vi "LVClass_WavefrontCorrectorSet Get Actions List.vi"(0 "WavefrontCorrectorSet in":refnum<class "WavefrontCorrectorSet.lvclass">, 11 "error in (no error)":errorcluster) -> (4 "WavefrontCorrectorSet out":refnum<class "WavefrontCorrectorSet.lvclass">, 6 "Actions list":string[](array[string]), 15 "error out":errorcluster)   [LabVIEW 2020, in "WavefrontCorrectorSet.lvclass"]
doc: "If parameter is a string to be selected among a finite set of strings, return\nthe size of this set. See Imop_WavefrontCorrectorSet_GetParameterOption.\n\n--------------------------------------------------------------------------------\n\n<B>wavefrontcorrector_setIn </B> : WavefrontCorrectorSet object.\n<B>wavefrontcorrector_setOut </B> : WavefrontCorrectorSet object.\n<B>parameter_name </B> : Parameter name.\n<B>size </B> : Size of the list (count of strings expected in that parameter).\n<B>ErrorIn </B> : Error\n<B>ErrorOut </B> : Error\n\n--------------------------------------------------------------------------------"
uses:
  WavefrontCorrectorSet.lvclass
  WavefrontCorrectorSet.lvclass/WavefrontCorrectorSet.ctl
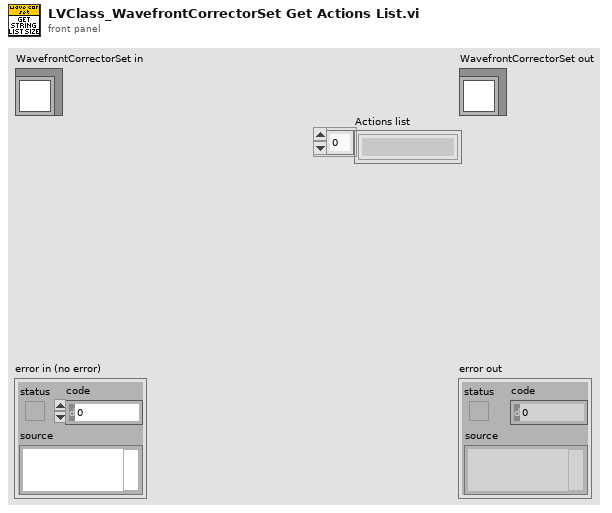
[diagram p1: front panel]
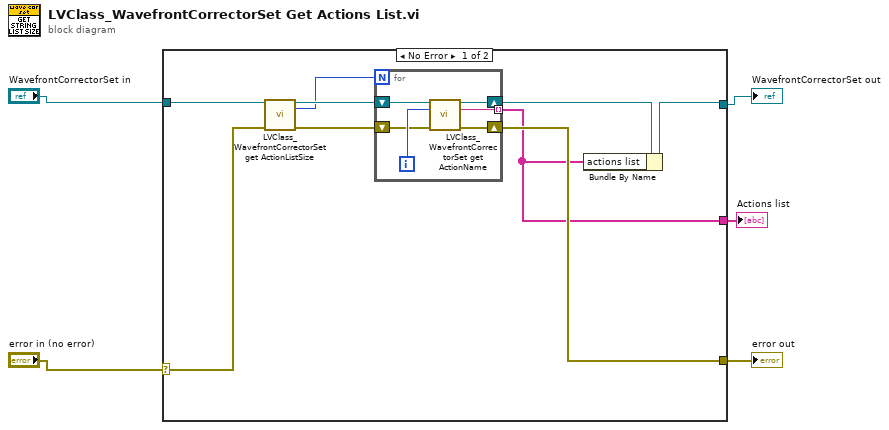
[diagram p0: block diagram]
diagram:
  n1 = case shown="No Error" "error in (no error)" {
    selector: "error in (no error)" -> [w11 w21]
    tunnel: "WavefrontCorrectorSet in" -> [w13 w22]
    tunnel: [w8 w22] -> w3
    tunnel: [w10 w21] -> w2
    tunnel: [w7 _] -> w1
    frame No Error {
      n2 = call "LVClass_WavefrontCorrectorSet get ActionListSize.vi"("WavefrontCorrectorSet in"=w13, "error in (no error)"=w11) -> ("WavefrontCorrectorSet out"=w14:refnum<class "WavefrontCorrectorSet.lvclass">, "ActionListSize"=w6:i32, "error out"=w12:errorcluster)  [unwired: 11 in]
      n3 = for {
        N: w6 -> [_]
        shift-right: [w18] -> w9
        shift-left: w14 -> [w20]
        shift-right: [w16] -> w10
        shift-left: w12 -> [w17]
        tunnel: [w15] -> w7 mode=indexing
        i -> [w19]
        n4 = call "LVClass_WavefrontCorrectorSet get ActionName.vi"("WavefrontCorrectorSet in"=w20, "index"=w19, "error in (no error)"=w17) -> ("WavefrontCorrectorSet out"=w18:refnum<class "WavefrontCorrectorSet.lvclass">, "Action Name"=w15:string, "error out"=w16:errorcluster)  [unwired: 10 in]
      }
      n5 = Bundle By Name(cluster=w9, "actions list"=w7) -> (w8:refnum<class "WavefrontCorrectorSet.lvclass">)
    }
    frame Error {
    }
  }
  "error out" <- w2
  "WavefrontCorrectorSet out" <- w3
  "Actions list" <- w1
